vi "Get Error.vi"(11 "Event Actor in":refnum<class "Event Actor.lvclass">) -> (2 "Error":errorcluster)   [LabVIEW 2021, in "Event Actor.lvclass"]
uses:
  Event Actor.lvclass
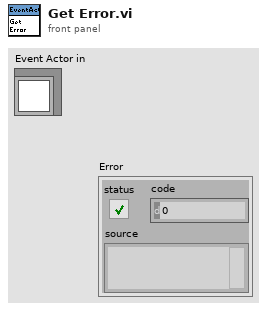
[diagram p1: front panel]
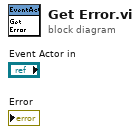
[diagram p0: block diagram]
diagram:
